vi "DebuggerTest.vi"() -> ()   [LabVIEW 2016]
uses:
  grsim/grSim Robot Command.ctl
  <extravilib>/ChannelInstances/Lossy Stream-a[.](u8)/Read With Abort.vi
  <extravilib>/ChannelInstances/Lossy Stream-a[.](u8)/Write With Abort.vi
  <extravilib>/ChannelInstances/Lossy Stream-a[.](u8)/Endpoint.vi
  <vilib>/Instr/_visa.llb/VISA Configure Serial Port (Instr).vi
  <extravilib>/ChannelInstances/Lossy Stream-a[.](u8)/Instantiate.vi
  <extravilib>/ChannelInstances/Lossy Stream-a[.](u8)/)Channel.vi
  <resource>/ChannelSupport/_ChannelSupport/WaitIfNeeded.vi
  <extravilib>/ChannelInstances/Lossy Stream-a[.](u8).lvlib
panel:
  in  "current sensor":bool
  in  "duty cycle 3":dbl format="%#_13g"
  out "Waveform Chart":sgl[][](graph)
  out "Robot cluster":T1
  in  "duty cycle 2":dbl format="%#_13g"
  in  "stop":bool
  in  "duty cycle":dbl format="%#_13g"
  in  "vel mtr":dbl[](array[numeric])
  in  "speed or step":bool
  in  "don´t plot":bool
  in  "plot":bool
  in  "K_D":dbl format="%#_13g"
  in  "K_I":dbl format="%#_13g"
  in  "K_P":dbl format="%#_13g"
  in  "pid":bool
  in  "motv 0":bool
  in  "*IDN?":bool
  out "spreadsheet string":string
  out "error out 2":errorcluster
  out "read buffer":string
  out "error out":errorcluster
  in  "termination char\n(0xA = '\\n' = LF)":u8=10 format="%.0x"
  in  "VISA resource name 2":refnum<visa-resource-name>
  in  "Serial Settings":T2={"baud rate"=9600, "data bits"=8, "parity"=enum."None", "stop bits"=10, "flow control"=0} {"flow control" items=["None"=0, "XON/XOFF"=1, "RTS/CTS"=2, "DTR/DSR"=4]; "stop bits" items=["1.0"=10, "1.5"=15, "2.0"=20]; "data bits" min=5 max=8 step=1; "baud rate" items=["75"=75, "110"=110, "134"=134, "150"=150, "300"=300, "600"=600, "1200"=1200, "1800"=1800, "2400"=2400, "4800"=4800, "7200"=7200, "9600"=9600, "14400"=14400, "19200"=19200, "28800"=28800, "38400"=38400, "56000"=56000, "57600"=57600, "115200"=115200, "128000"=128000, "230400"=230400]}
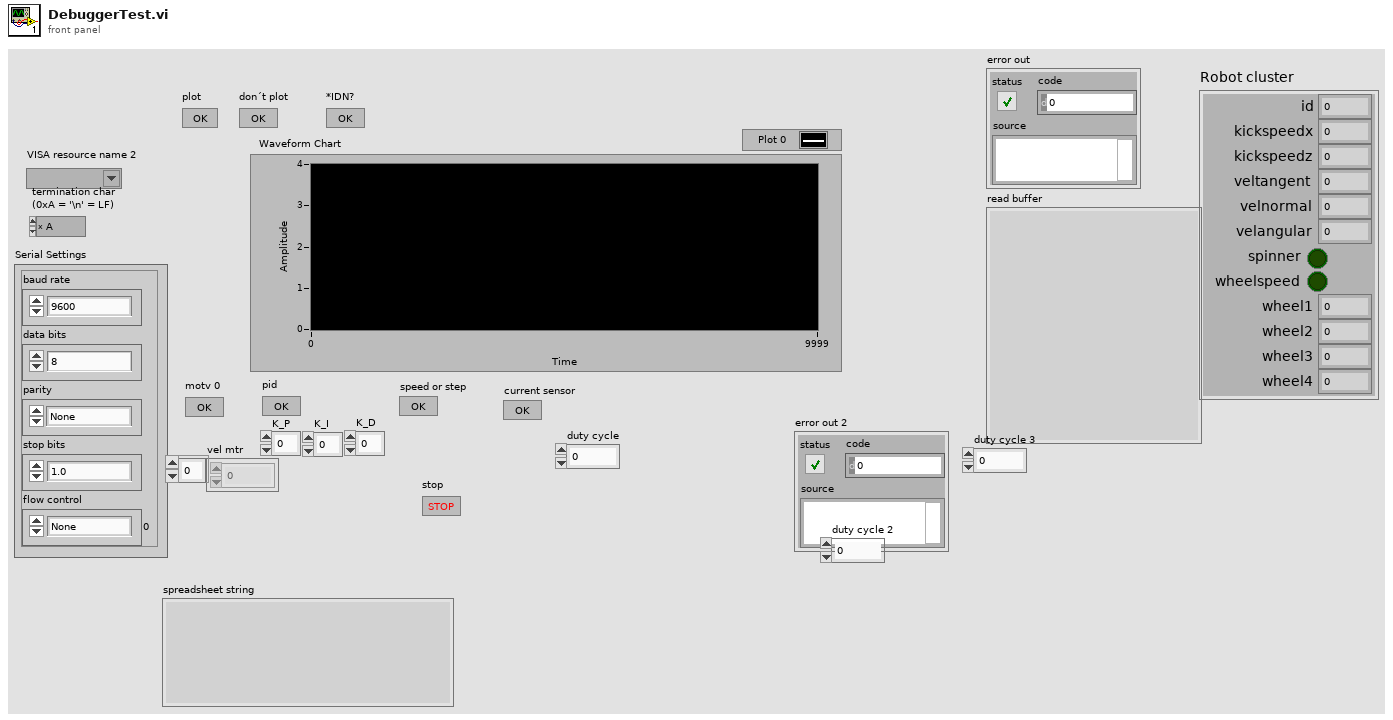
[diagram p1: front panel]
types:
  T1 = typedef "grSim Robot Command.ctl" = cluster{"id":u32, "kickspeedx":sgl, "kickspeedz":sgl, "veltangent":sgl, "velnormal":sgl, "velangular":sgl, "spinner":bool, "wheelspeed":bool, "wheel1":sgl, "wheel2":sgl, "wheel3":sgl, "wheel4":sgl}
  T2 = cluster{"baud rate":u32, "data bits":u16, "parity":enum16{"None", "Odd", "Even", "Mark", "Space"}, "stop bits":u16, "flow control":u16}
  T3 = typedef "Lossy Stream-a[.](u8).lvlib/)Channel.ctl" = refnum<queue>
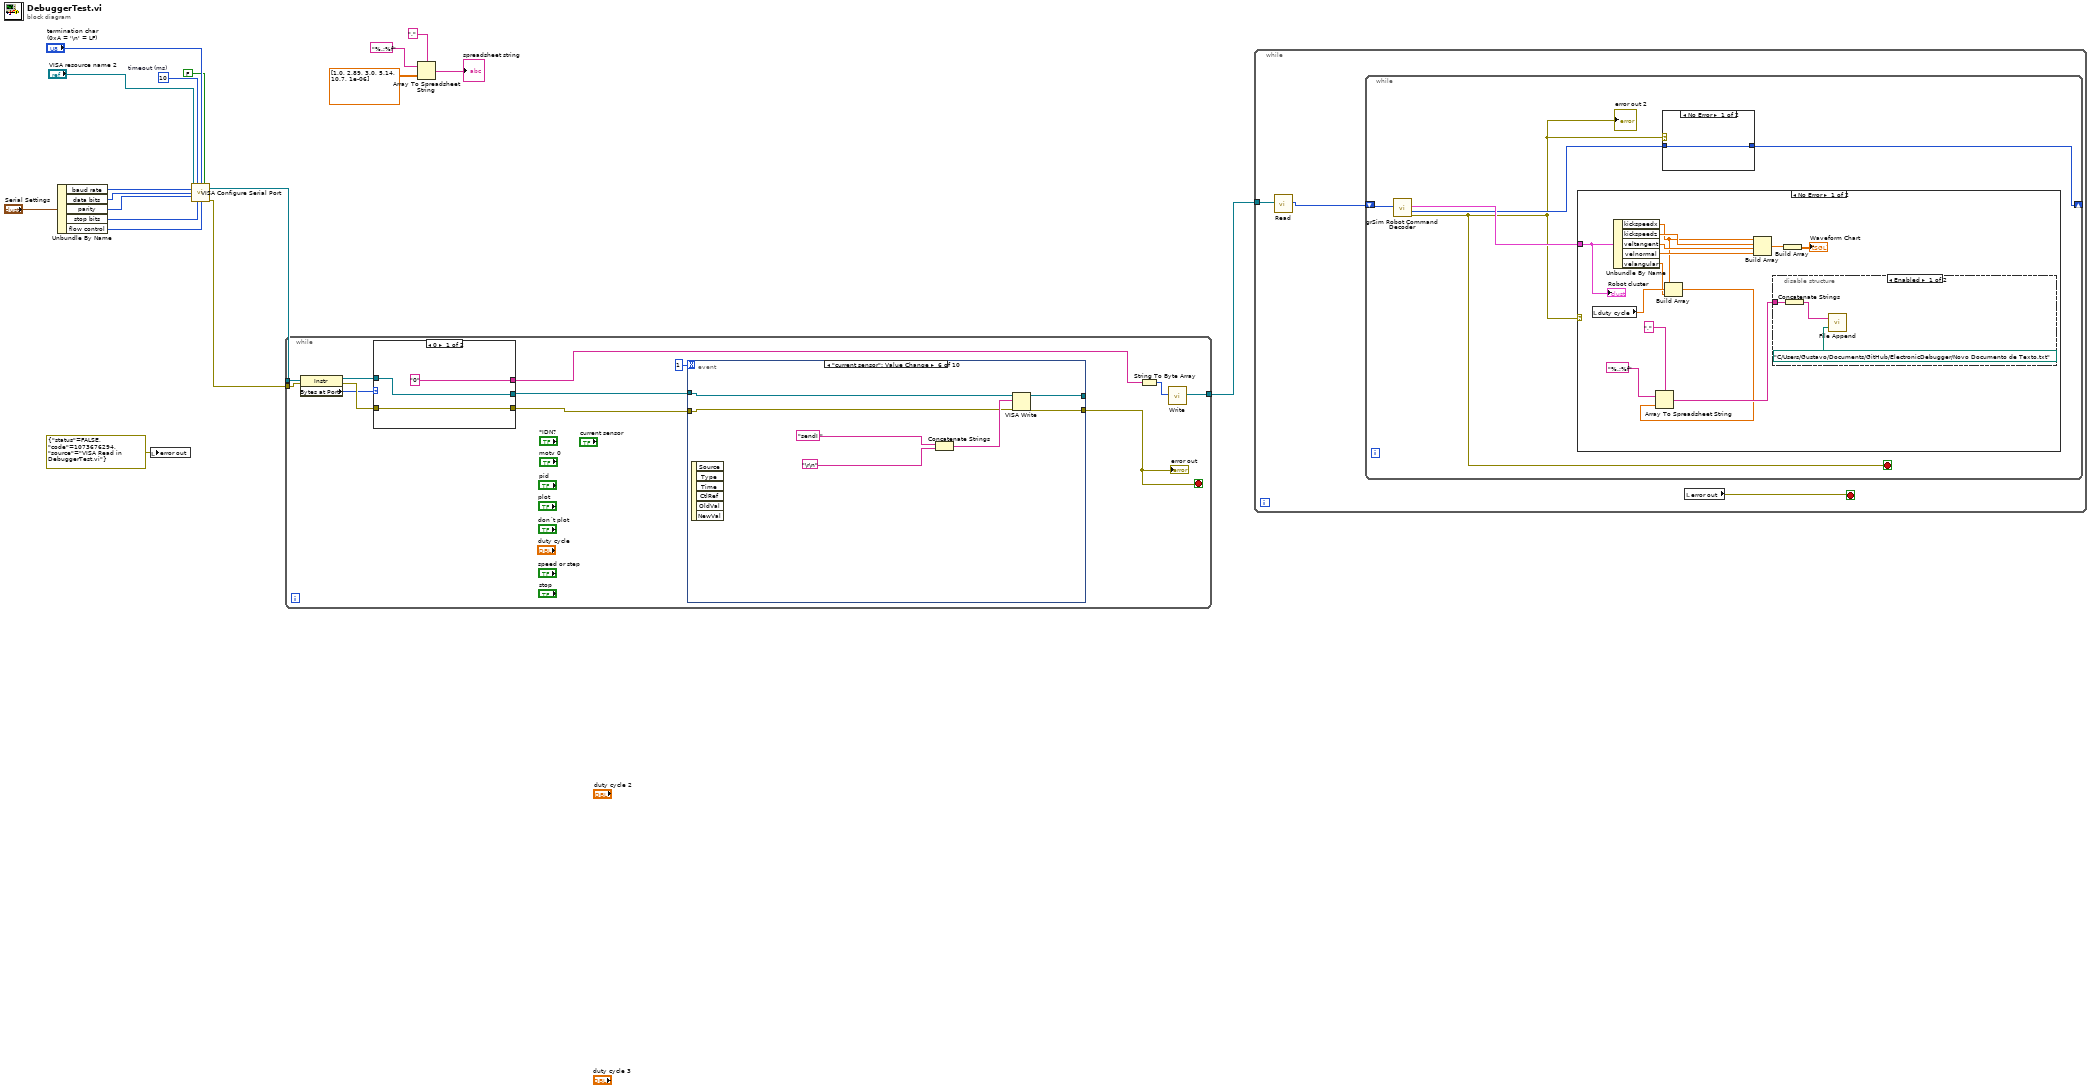
[diagram p0: block diagram]
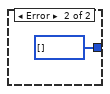
[diagram p4: hidden frame]
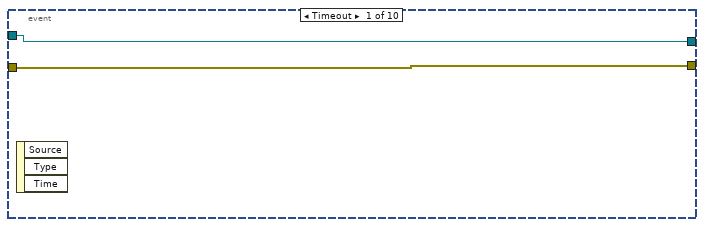
[diagram p5: hidden frame]
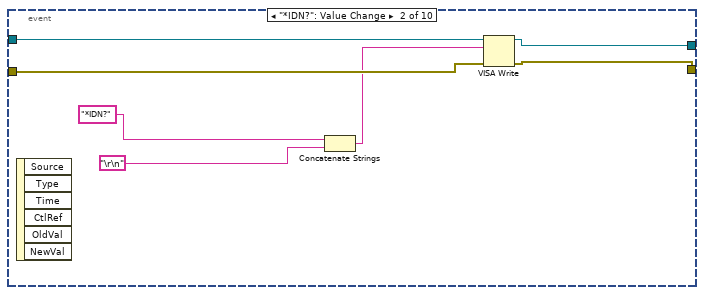
[diagram p6: hidden frame]
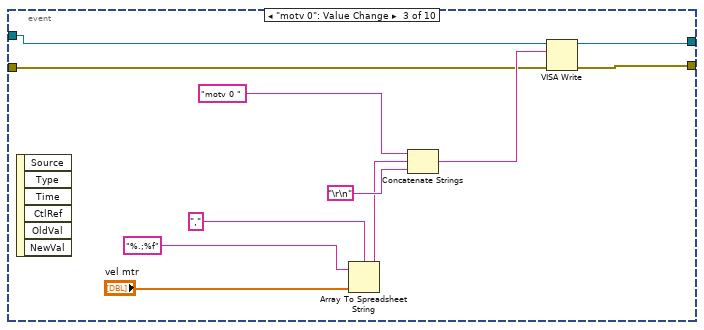
[diagram p7: hidden frame]
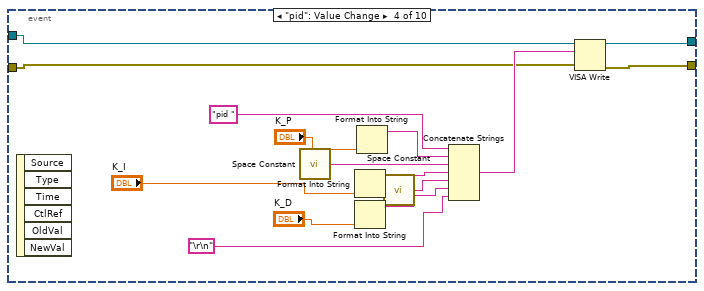
[diagram p8: hidden frame]
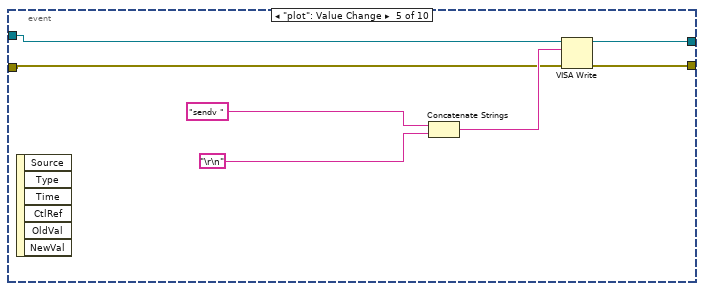
[diagram p9: hidden frame]
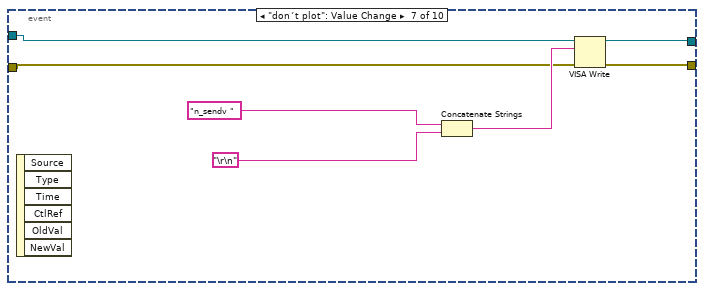
[diagram p10: hidden frame]
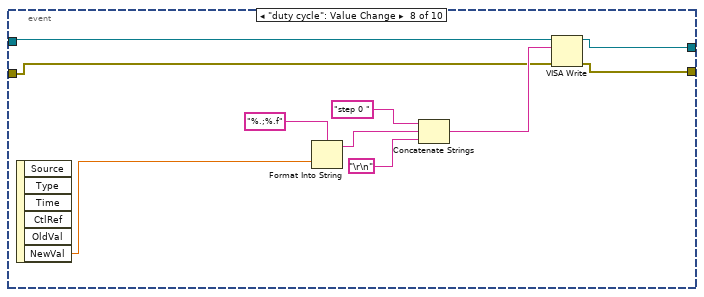
[diagram p11: hidden frame]
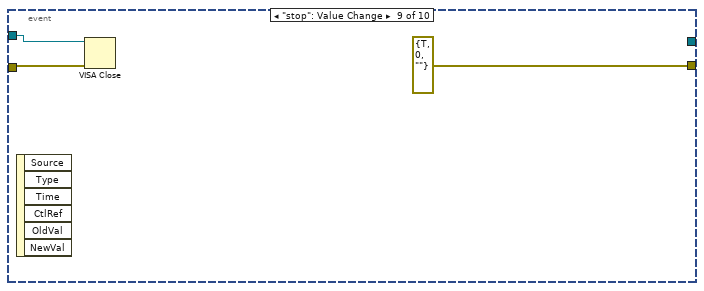
[diagram p12: hidden frame]
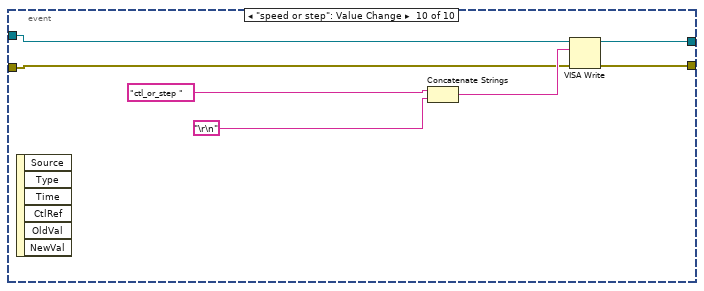
[diagram p13: hidden frame]
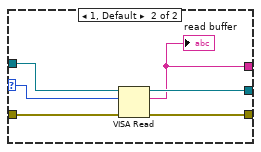
[diagram p14: hidden frame]
diagram:
  w9 = u32 10  # timeout (ms)
  n1 = Unbundle By Name("Serial Settings") -> ("baud rate"=w17:u32, "data bits"=w16:u16, "parity"=w15:enum16{"None", "Odd", "Even", "Mark", "Space"}, "stop bits"=w14:u16, "flow control"=w13:u16)
  n2 = local write "error out"(errorcluster {"status"=FALSE, "code"=1073676294, "source"="VISA Read in DebuggerTest.vi"} ("error out")) -> ()
  n3 = call-poly "VISA Configure Serial Port"("VISA resource name"="VISA resource name 2", "timeout (10sec)"=w9, "termination char\n(0xA = '\\n' = LF)"="termination char\n(0xA = '\\n' = LF)", "Enable Termination\nChar (T)"=FALSE ("Enable Termination\nChar (T)"), "baud rate (9600)"=w17, "data bits (8)"=w16, "parity (0:none)"=w15, "stop bits (10: 1 bit)"=w14, "flow control (0:none)"=w13) -> ("VISA resource name out"=w8:refnum<visa-resource-name>, "error out"=w7:errorcluster)  [unwired: 5 in]
  n4 = while {
    tunnel: w8 -> [w30]
    tunnel: [w28] -> w6
    tunnel: w7 -> [w27]
    stop <- w19 stop-if-true
    n5 = property class="Instr"(reference=w30, error in=w27) -> (reference out=w29:refnum<visa-resource-name>, error out=w26:errorcluster, "Bytes at Port"=w24:u32)
    n6 = case shown="0" w24 {
      selector: w24 -> [_ w111]
      tunnel: w29 -> [w108 w115]
      tunnel: w26 -> [w109 w114]
      tunnel: [w108 w113] -> w23
      tunnel: ["0" ("read buffer") w110] -> w21
      tunnel: [w109 w112] -> w22
      frame 0 {
      }
      frame 1, Default {
        n7 = VISA Read(VISA resource name=w115, byte count=w111, error in (no error)=w114) -> (VISA resource name out=w113:refnum<visa-resource-name>, read buffer=w110:string, error out=w112:errorcluster)  [unwired: 1 out]
        "read buffer" <- w110
      }
    }
    n8 = event shown="[5] \"current sensor\": Value Change" {
      selector: _ -> [_ _ _ _ _ _ _ _ _ _]
      dyn-events: _ -> [_ _ _ _ _ _ _ _ _ _]
      timeout: 1 -> [_ _ _ _ _ _ _ _ _ _]
      tunnel: w23 -> [w31 w39 w48 w61 w69 w76 w82 w91 w98 w104]
      tunnel: w22 -> [w32 w38 w47 w62 w70 w75 w81 w90 w97 w103]
      tunnel: [w32 w37 w45 w63 w68 w73 w83 w88 errorcluster {"status"=TRUE, "code"=0, "source"=""} ("error out") w102] -> w19
      tunnel: [w31 w33 w44 w51 w66 w74 w80 w89 _ w100] -> _
      event Timeout {
        n9 = event-data() -> ()  [unwired: 1 in, 3 out]
      }
      event "*IDN?": Value Change {
        n10 = event-data() -> ()  [unwired: 1 in, 6 out]
        n11 = Concatenate Strings("*IDN?" ("write buffer"), "\r\n") -> (w36:string)
        n12 = VISA Write(VISA resource name=w39, write buffer=w36, error in (no error)=w38) -> (VISA resource name out=w33:refnum<visa-resource-name>, error out=w37:errorcluster)  [unwired: 1 out]
      }
      event "motv 0": Value Change {
        n13 = event-data() -> ()  [unwired: 1 in, 6 out]
        n14 = Array To Spreadsheet String(delimiter (Tab)=",", array="vel mtr", 3:"%.;%f" ("format string")) -> (spreadsheet string=w40:string)
        n15 = Concatenate Strings("motv 0 " ("write buffer"), w40, "\r\n") -> (w49:string)
        n16 = VISA Write(VISA resource name=w48, write buffer=w49, error in (no error)=w47) -> (VISA resource name out=w44:refnum<visa-resource-name>, error out=w45:errorcluster)  [unwired: 1 out]
      }
      event "pid": Value Change {
        n17 = event-data() -> ()  [unwired: 1 in, 6 out]
        n18 = call <vilib>:"Space Constant.vi"() -> ("String"=w56:string)
        n19 = Format Into String("K_I") -> (resulting string=w55:string)  [unwired: 3 in, 1 out]
        n20 = Format Into String("K_D") -> (resulting string=w53:string)  [unwired: 3 in, 1 out]
        n21 = Format Into String("K_P") -> (resulting string=w57:string)  [unwired: 3 in, 1 out]
        n22 = call <vilib>:"Space Constant.vi"() -> ("String"=w54:string)
        n23 = Concatenate Strings("pid " ("write buffer"), w57, w56, w55, w54, w53, "\r\n") -> (w65:string)
        n24 = VISA Write(VISA resource name=w61, write buffer=w65, error in (no error)=w62) -> (VISA resource name out=w51:refnum<visa-resource-name>, error out=w63:errorcluster)  [unwired: 1 out]
      }
      event "plot": Value Change {
        n25 = event-data() -> ()  [unwired: 1 in, 6 out]
        n26 = Concatenate Strings("sendv " ("write buffer"), "\r\n") -> (w72:string)
        n27 = VISA Write(VISA resource name=w69, write buffer=w72, error in (no error)=w70) -> (VISA resource name out=w66:refnum<visa-resource-name>, error out=w68:errorcluster)  [unwired: 1 out]
      }
      event "current sensor": Value Change {
        n28 = event-data() -> ()  [unwired: 1 in, 6 out]
        n29 = Concatenate Strings("sendI " ("write buffer"), "\r\n") -> (w79:string)
        n30 = VISA Write(VISA resource name=w76, write buffer=w79, error in (no error)=w75) -> (VISA resource name out=w74:refnum<visa-resource-name>, error out=w73:errorcluster)  [unwired: 1 out]
      }
      event "don´t plot": Value Change {
        n31 = event-data() -> ()  [unwired: 1 in, 6 out]
        n32 = Concatenate Strings("n_sendv " ("write buffer"), "\r\n") -> (w84:string)
        n33 = VISA Write(VISA resource name=w82, write buffer=w84, error in (no error)=w81) -> (VISA resource name out=w80:refnum<visa-resource-name>, error out=w83:errorcluster)  [unwired: 1 out]
      }
      event "duty cycle": Value Change {
        n34 = event-data() -> ("NewVal"=w87:dbl)  [unwired: 1 in, 5 out]
        n35 = Format Into String(format string="%.;%.f", w87) -> (resulting string=w93:string)  [unwired: 2 in, 1 out]
        n36 = Concatenate Strings("step 0 " ("write buffer"), w93, "\r\n") -> (w96:string)
        n37 = VISA Write(VISA resource name=w91, write buffer=w96, error in (no error)=w90) -> (VISA resource name out=w89:refnum<visa-resource-name>, error out=w88:errorcluster)  [unwired: 1 out]
      }
      event "stop": Value Change {
        n38 = event-data() -> ()  [unwired: 1 in, 6 out]
        n39 = VISA Close(VISA resource name=w98, error in (no error)=w97) -> ()  [unwired: 1 out]
      }
      event "speed or step": Value Change {
        n40 = event-data() -> ()  [unwired: 1 in, 6 out]
        n41 = Concatenate Strings("ctl_or_step " ("write buffer"), "\r\n") -> (w105:string)
        n42 = VISA Write(VISA resource name=w104, write buffer=w105, error in (no error)=w103) -> (VISA resource name out=w100:refnum<visa-resource-name>, error out=w102:errorcluster)  [unwired: 1 out]
      }
    }
    "error out" <- w19
    n43 = String To Byte Array(string=w21) -> (unsigned byte array=w25:u8[])
    n44 = call <extravilib>:"Write.vi"("element"=w25) -> ("channel"=w28:T3)  [unwired: 8 in, 2 out]
  }
  n45 = Array To Spreadsheet String(delimiter (Tab)=",", array=dbl[][] [[1.0, 2.89], [3.0, 5.14], [10.7, 1e-06]], 3:"%.;%f" ("format string")) -> (spreadsheet string=→"spreadsheet string":string)
  n46 = while {
    tunnel: w6 -> [w118]
    stop <- w117 stop-if-true
    n47 = call <extravilib>:"Read.vi"("channel"=w118) -> ("element"=w116:u8[])  [unwired: 5 in, 5 out]
    n48 = while {
      shift-right: [w119] -> _
      shift-left: w116 -> [w120]
      stop <- w121 stop-if-true
      n49 = call "grSim Robot Command Decoder.vi"("Array"=w120) -> ("error out"=w121:errorcluster, "array w/ subset deleted"=w122:u8[], "Robot cluster"=w123:T1)  [unwired: 8 in]
      "error out 2" <- w121
      n50 = case shown="No Error" w121 {
        tunnel: w123 -> [w124 _]
        frame No Error {
          n51 = local read "duty cycle"() -> (w126:dbl)
          n52 = Unbundle By Name(w124) -> ("kickspeedx"=w128:sgl, "kickspeedz"=w136:sgl, "veltangent"=w135:sgl, "velnormal"=w134:sgl, "velangular"=w125:sgl)
          n53 = Build Array(w128, w126, w125) -> (w127:dbl[])
          n54 = Array To Spreadsheet String(delimiter (Tab)=",", array=w127, 3:"%.;%f" ("format string")) -> (spreadsheet string=w129:string)
          n55 = Build Array(w128, w136, w135, w134) -> (w133:sgl[])
          n56 = disable-structure shown="Enabled" {
            disable-tunnel: w129 -> [w137 _]
            frame Enabled {
              n57 = Concatenate Strings(w137) -> (w138:string)
              n58 = call "File Append.vi"("file path"=path "C:/Users/Gustavo/Documents/GitHub/ElectronicDebugger/Novo Documento de Texto.txt", "String"=w138) -> ()  [unwired: 2 in]
            }
            frame Disabled {
            }
          }
          n59 = Build Array(w133) -> (→"Waveform Chart":sgl[][])
          "Robot cluster" <- w124
        }
        frame Error {
        }
      }
      n60 = case shown="No Error" w121 {
        tunnel: w122 -> [w140 _]
        tunnel: [w140 u8[] [] ("array w/ subset deleted")] -> w119
        frame No Error {
        }
        frame Error {
        }
      }
    }
    n61 = local read "error out"() -> (w117:errorcluster)
  }
